vi "실습 2-4 링컨트롤.vi"() -> ()   [LabVIEW 2014]
panel:
  out "초 단위":dbl
  in  "시간입력":dbl=1.2
  in  "링":u32(ring)=1 items=["초"=1, "분"=60, "시간"=3600, "일"=86400]
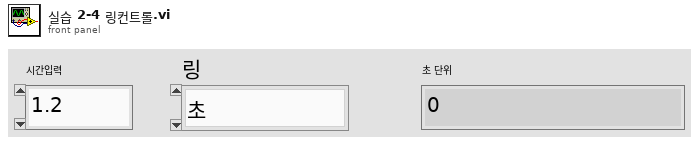
[diagram p1: front panel]
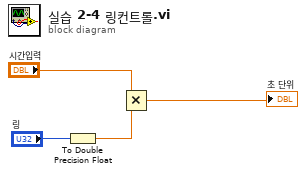
[diagram p0: block diagram]
diagram:
  n1 = To Double Precision Float(number="링") -> (double precision float=w2:dbl)
  n2 = Multiply(x="시간입력", y=w2) -> (x*y=→"초 단위":dbl)
